vi "Calculate New Thermistor Calibrations.vi"(7 "Manifold Ambient Temperature":dbl=nan format="%#_14g", 8 "error in":errorcluster, 9 "Therm_Offset":i32=-1, 10 "Therm_Input":i32=-1, 11 "Therm_Bias":i32=-1) -> (0 "error out":errorcluster, 1 "Cal Abort Threshold (R/4)":string="NaN", 2 "Cal Critical Threshold (R/4)":string="NaN", 3 "Cal Warning Threshold (R/4)":string="NaN", 5 "Cal Minimum Threshold (R/4)":string="NaN")   [LabVIEW 2010]
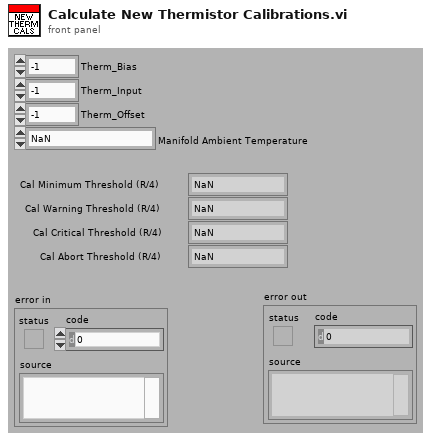
[diagram p1: front panel]
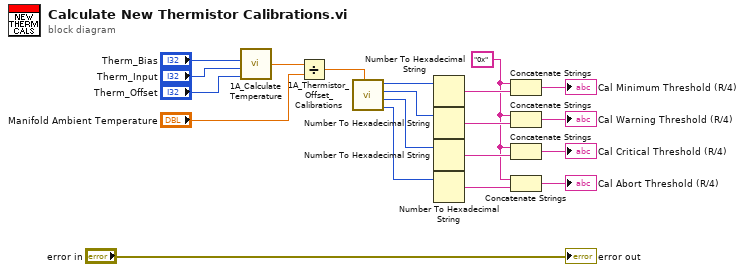
[diagram p0: block diagram]
diagram:
  w1 = "0x" ("string")
  n1 = call "1A_Calculate Temperature.vi"("Therm_Offset"="Therm_Offset", "Therm_Input"="Therm_Input", "Therm_Bias"="Therm_Bias") -> ("Temperature"=w17:dbl)  [unwired: 2 in, 1 out]
  n2 = Divide(x=w17, y="Manifold Ambient Temperature") -> (x/y=w15:dbl)
  n3 = call "1A_Thermistor_Offset_Calibrations.vi"("Offset Ratio"=w15) -> ("Cal Abort Threshold (R/4)"=w11:u16, "Cal Critical Threshold (R/4)"=w12:u16, "Cal Warning Threshold (R/4)"=w13:u16, "Cal Minimum Threshold (R/4)"=w14:u16)  [unwired: 7 in]
  n4 = Number To Hexadecimal String(2:w14) -> (0:w9:string)  [unwired: 1 in]
  n5 = Number To Hexadecimal String(2:w13) -> (0:w7:string)  [unwired: 1 in]
  n6 = Number To Hexadecimal String(2:w12) -> (0:w6:string)  [unwired: 1 in]
  n7 = Number To Hexadecimal String(2:w11) -> (0:w5:string)  [unwired: 1 in]
  n8 = Concatenate Strings(w1, w9) -> (→"Cal Minimum Threshold (R/4)":string)
  n9 = Concatenate Strings(w1, w7) -> (→"Cal Warning Threshold (R/4)":string)
  n10 = Concatenate Strings(w1, w6) -> (→"Cal Critical Threshold (R/4)":string)
  n11 = Concatenate Strings(w1, w5) -> (→"Cal Abort Threshold (R/4)":string)
  "error out" <- "error in"
